vi "评估局面.vi"(1 "输入的棋盘":T1) -> (0 "优势程度":dbl)   [LabVIEW 2017]
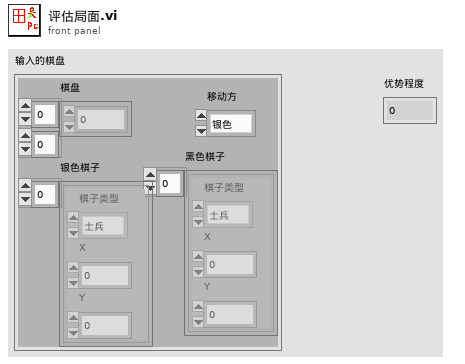
[diagram p1: front panel]
types:
  T1 = cluster{"棋盘":u16[][], "银色棋子":cluster{"棋子类型":enum16{"士兵", "骑士", "主教", "战车", "皇后", "国王", "空"}, "X":u8, "Y":u8}[], "黑色棋子":cluster{"棋子类型":enum16{"士兵", "骑士", "主教", "战车", "皇后", "国王", "空"}, "X":u8, "Y":u8}[], "移动方":enum16{"银色", "黑色"}}
  T2 = cluster{"棋子类型":enum16{"士兵", "骑士", "主教", "战车", "皇后", "国王", "空"}, "X":u8, "Y":u8}[]
  T3 = cluster{"棋子类型":enum16{"士兵", "骑士", "主教", "战车", "皇后", "国王", "空"}, "X":u8, "Y":u8}
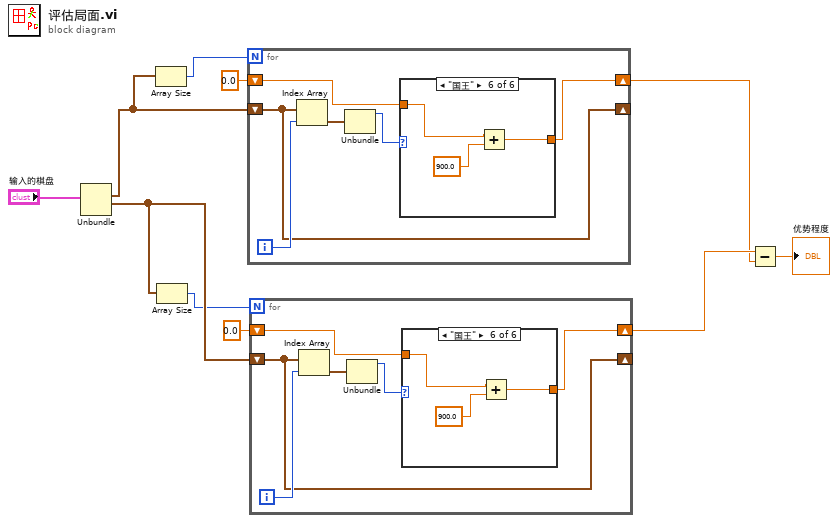
[diagram p0: block diagram]
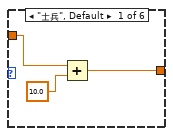
[diagram p2: hidden frame]
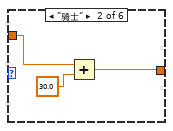
[diagram p3: hidden frame]
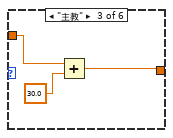
[diagram p4: hidden frame]
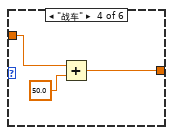
[diagram p5: hidden frame]
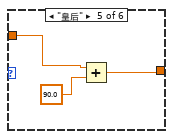
[diagram p6: hidden frame]
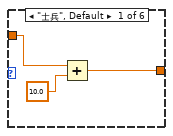
[diagram p7: hidden frame]
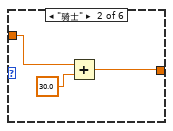
[diagram p8: hidden frame]
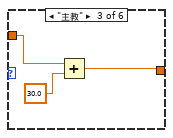
[diagram p9: hidden frame]
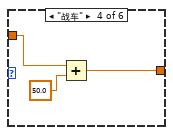
[diagram p10: hidden frame]
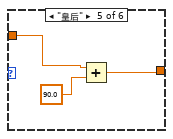
[diagram p11: hidden frame]
diagram:
  n1 = Unbundle("输入的棋盘") -> ("银色棋子"=w8:T2, "黑色棋子"=w6:T2)  [unwired: 2 out]
  n2 = Array Size(array=w8) -> (size(s)=w7:i32)
  n3 = Array Size(array=w6) -> (size(s)=w5:i32)
  n4 = for {
    N: w7 -> [_]
    shift-right: [w11] -> _
    shift-left: w8 -> [w11]
    shift-right: [w12] -> w2
    shift-left: 0.0 -> [w13]
    i -> [w16]
    n5 = Index Array(array=w11, index=w16) -> (element=w15:T3)
    n6 = Unbundle(w15) -> ("棋子类型"=w14:enum16{"士兵", "骑士", "主教", "战车", "皇后", "国王", "空"})  [unwired: 2 out]
    n7 = case shown="\"国王\"" w14 {
      tunnel: w13 -> [w19 w21 w25 w27 w30 w33]
      tunnel: [w17 w20 w23 w28 w31 w34] -> w12
      frame "士兵", Default {
        n8 = Add(x=w19, y=10.0) -> (x+y=w17:dbl)
      }
      frame "骑士" {
        n9 = Add(x=w21, y=30.0) -> (x+y=w20:dbl)
      }
      frame "主教" {
        n10 = Add(x=w25, y=30.0) -> (x+y=w23:dbl)
      }
      frame "战车" {
        n11 = Add(x=w27, y=50.0) -> (x+y=w28:dbl)
      }
      frame "皇后" {
        n12 = Add(x=w30, y=90.0) -> (x+y=w31:dbl)
      }
      frame "国王" {
        n13 = Add(x=w33, y=900.0) -> (x+y=w34:dbl)
      }
    }
  }
  n14 = for {
    N: w5 -> [_]
    shift-right: [w35] -> _
    shift-left: w6 -> [w35]
    shift-right: [w36] -> w3
    shift-left: 0.0 -> [w37]
    i -> [w40]
    n15 = Index Array(array=w35, index=w40) -> (element=w39:T3)
    n16 = Unbundle(w39) -> ("棋子类型"=w38:enum16{"士兵", "骑士", "主教", "战车", "皇后", "国王", "空"})  [unwired: 2 out]
    n17 = case shown="\"国王\"" w38 {
      tunnel: w37 -> [w43 w45 w49 w51 w54 w57]
      tunnel: [w41 w44 w47 w52 w55 w58] -> w36
      frame "士兵", Default {
        n18 = Add(x=w43, y=10.0) -> (x+y=w41:dbl)
      }
      frame "骑士" {
        n19 = Add(x=w45, y=30.0) -> (x+y=w44:dbl)
      }
      frame "主教" {
        n20 = Add(x=w49, y=30.0) -> (x+y=w47:dbl)
      }
      frame "战车" {
        n21 = Add(x=w51, y=50.0) -> (x+y=w52:dbl)
      }
      frame "皇后" {
        n22 = Add(x=w54, y=90.0) -> (x+y=w55:dbl)
      }
      frame "国王" {
        n23 = Add(x=w57, y=900.0) -> (x+y=w58:dbl)
      }
    }
  }
  n24 = Subtract(x=w3, y=w2) -> (x-y=→"优势程度":dbl)
